vi "Low Pass Differentiator.vi"(8 "Smoothing Factor":dbl=0.1, 10 "dt":dbl, 11 "X":dbl) -> (3 "dX, smoothed":dbl)   [LabVIEW 2011]
doc: "Differentiates the input and applies exponential smoothing to the output. Exponential smoothing weights the input value (in this case, the differentiated value) against the previous smoothing value."
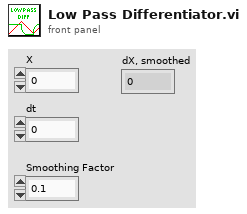
[diagram p1: front panel]
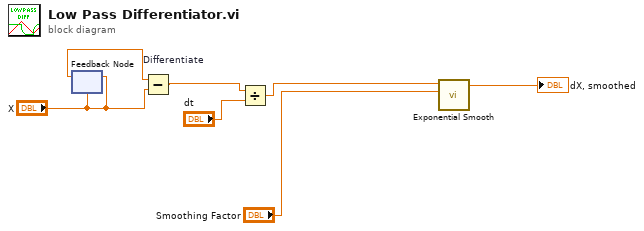
[diagram p0: block diagram]
diagram:
  n1 = feedback #1("X") -> (w6:dbl)
  n2 = feedback-in #1("X") -> ()
  n3 = Subtract "Differentiate"(x=w6, y="X") -> (x-y=w3:dbl)
  n4 = Divide(x=w3, y="dt") -> (x/y=w1:dbl)
  n5 = call "Exponential Smooth.vi"("Smoothing Factor"="Smoothing Factor", "Input Value"=w1) -> ("Smoothed Value"=→"dX, smoothed":dbl)  [unwired: 9 in]
